vi "UseDeviceKey (with Device VIs).vi"() -> ()   [LabVIEW 2009]
panel:
  out "Device Count":i32
  out "Device Keys Out":string[](array[string])
  out "Output:":string
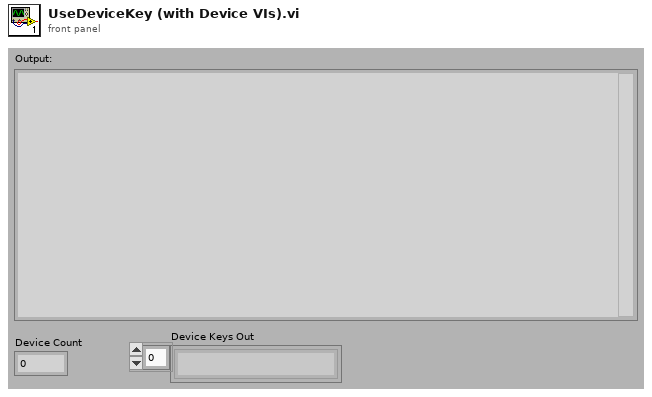
[diagram p1: front panel]
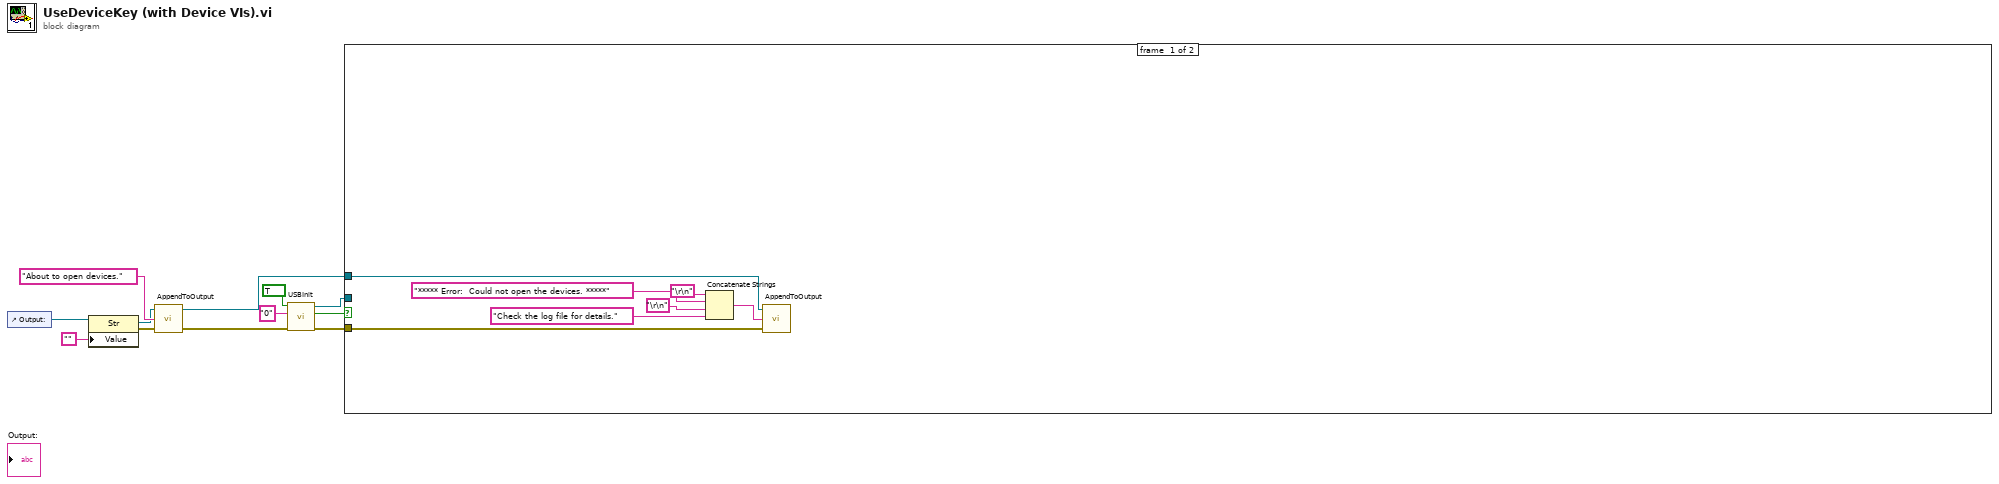
[diagram p0: block diagram]
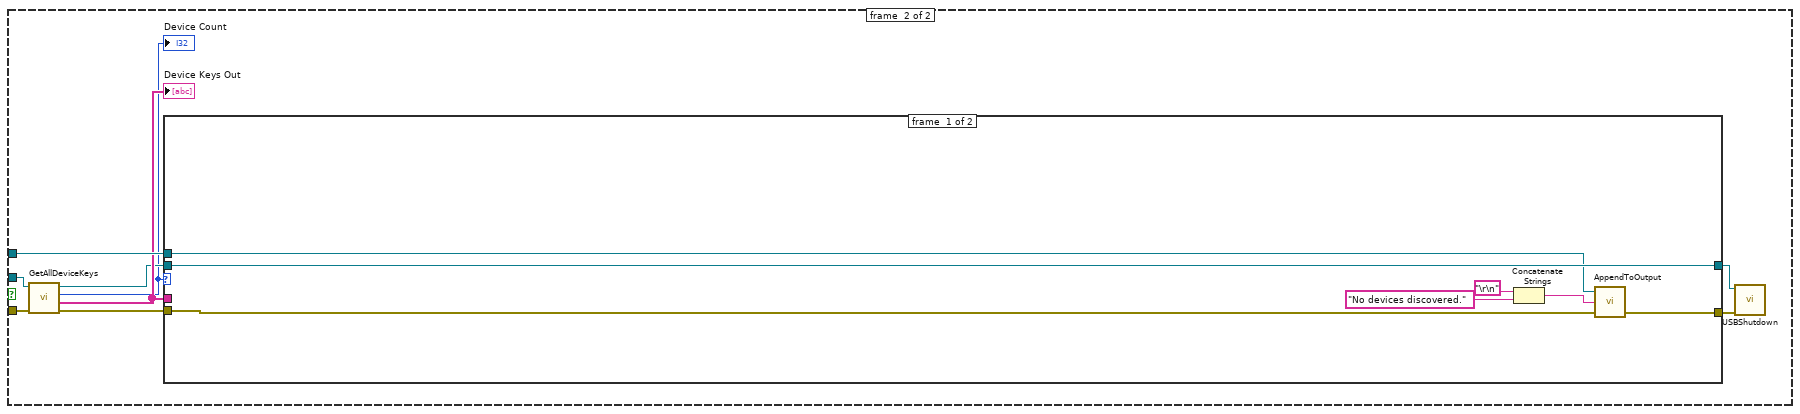
[diagram p2: hidden frame]
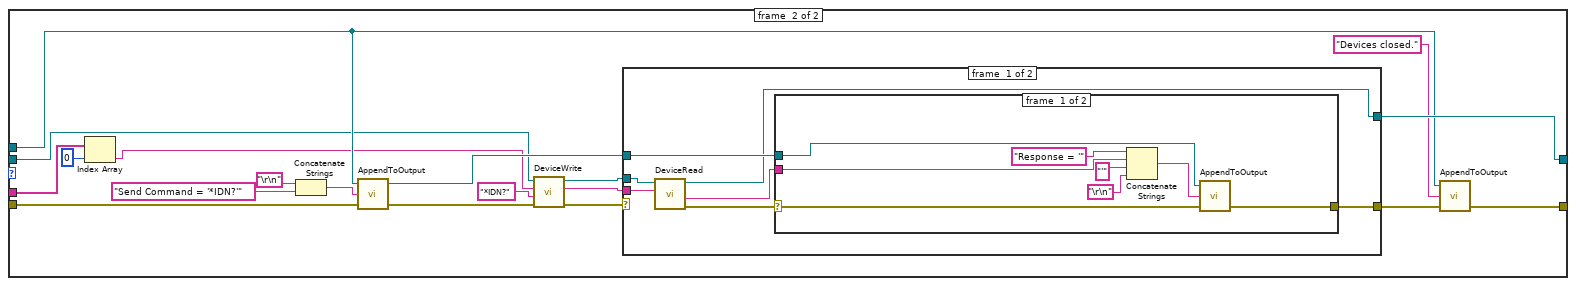
[diagram p3: hidden frame]
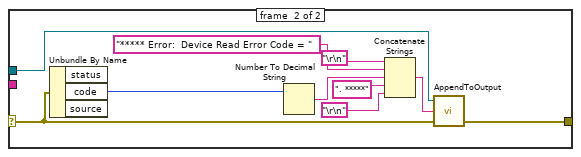
[diagram p4: hidden frame]
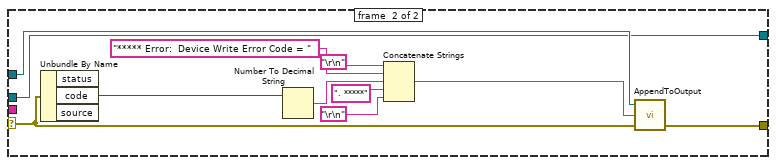
[diagram p5: hidden frame]
diagram:
  n1 = control-ref of="Output:"() -> (w10:refnum<vi>)
  n2 = property class="Str"(reference=w10, "Value"="") -> (reference out=w7:refnum<vi>, error out=w8:errorcluster)  [unwired: 1 in]
  n3 = call "AppendToOutput.vi"("error in"=w8, "Input String"="About to open devices.", "Output Refnum In"=w7) -> ("error out"=w4:errorcluster, "Output Refnum Out"=w11:refnum<vi>)  [unwired: 1 in]
  n4 = call "USBInit.vi"("error in (no error)"=w4, "Product ID"="0", "logging"=TRUE) -> ("error out"=w2:errorcluster, "Pass-Fail Status"=w3:bool, "USBLib Out"=w1:refnum<k24>)  [unwired: 2 in]
  n5 = case shown="True" w3 {
    tunnel: w11 -> [w19 w24]
    tunnel: w2 -> [w18 w25]
    tunnel: w1 -> [_ w26]
    frame #0 {
      n6 = Concatenate Strings("\r\n", "***** Error:  Could not open the devices. *****", "\r\n", "Check the log file for details.") -> (w14:string)
      n7 = call "AppendToOutput.vi"("error in"=w18, "Input String"=w14, "Output Refnum In"=w19) -> ()  [unwired: 1 in, 2 out]
    }
    frame #1 {
      n8 = call "GetAllDeviceKeys.vi"("error in (no error)"=w25, "USBLib In"=w26) -> ("error out"=w21:errorcluster, "Device Keys Out"=w23:string[], "Device Count"=w20:i32, "USBLib Out"=w22:refnum<k24>)  [unwired: 6 in]
      "Device Keys Out" <- w23
      "Device Count" <- w20
      n9 = case shown="1, Default" w20 {
        tunnel: [w32 w52] -> w28
        tunnel: [w35 w51] -> w27
        tunnel: w24 -> [w34 w50]
        tunnel: w23 -> [_ w44]
        tunnel: w22 -> [w35 w41]
        tunnel: w21 -> [w33 w40]
        frame #0 {
          n10 = Concatenate Strings("\r\n", "No devices discovered." ("Input String")) -> (w29:string)
          n11 = call "AppendToOutput.vi"("error in"=w33, "Input String"=w29, "Output Refnum In"=w34) -> ("error out"=w32:errorcluster)  [unwired: 1 in, 1 out]
        }
        frame #1 {
          n12 = Index Array(array=w44, index=0) -> (element=w42:string)
          n13 = Concatenate Strings("\r\n", "Send Command = '*IDN?'") -> (w36:string)
          n14 = call "AppendToOutput.vi"("error in"=w40, "Input String"=w36, "Output Refnum In"=w50) -> ("error out"=w49:errorcluster, "Output Refnum Out"=w54:refnum<vi>)  [unwired: 1 in]
          n15 = call "DeviceWrite.vi"("error in (no error)"=w49, "Command"="*IDN?" ("cmd"), "DeviceKey In"=w42, "USBLib In"=w41) -> ("error out"=w45:errorcluster, "DeviceKey Out"=w47:string, "USBLib Out"=w46:refnum<k24>)  [unwired: 1 in]
          n16 = case shown="No Error" w45 {
            selector: w45 -> [_ w81]
            tunnel: [w61 w84] -> w53
            tunnel: w54 -> [w60 w83]
            tunnel: w47 -> [w57 _]
            tunnel: [w59 w80] -> w51
            tunnel: w46 -> [w58 w80]
            frame #0 {
              n17 = call "DeviceRead.vi"("DeviceKey In"=w57, "USBLib In"=w58) -> ("error out"=w56:errorcluster, "Response"=w55:string, "USBLib Out"=w59:refnum<k24>)  [unwired: 2 in, 1 out]
              n18 = case shown="No Error" w56 {
                selector: w56 -> [w62 w70]
                tunnel: [w65 w72] -> w61
                tunnel: w60 -> [w64 w73]
                tunnel: w55 -> [w63 _]
                frame #0 {
                  n19 = Concatenate Strings("Response = '", w63, "'", "\r\n") -> (w66:string)
                  n20 = call "AppendToOutput.vi"("error in"=w62, "Input String"=w66, "Output Refnum In"=w64) -> ("error out"=w65:errorcluster)  [unwired: 1 in, 1 out]
                }
                frame #1 {
                  n21 = Unbundle By Name(w70) -> ("code"=w71:i32)  [unwired: 2 out]
                  n22 = Number To Decimal String(number=w71) -> (decimal integer string=w79:string)  [unwired: 1 in]
                  n23 = Concatenate Strings("\r\n", "***** Error:  Device Read Error Code = ", w79, ". *****", "\r\n") -> (w74:string)
                  n24 = call "AppendToOutput.vi"("error in"=w70, "Input String"=w74, "Output Refnum In"=w73) -> ("error out"=w72:errorcluster)  [unwired: 1 in, 1 out]
                }
              }
            }
            frame #1 {
              n25 = Unbundle By Name(w81) -> ("code"=w82:i32)  [unwired: 2 out]
              n26 = Number To Decimal String(number=w82) -> (decimal integer string=w86:string)  [unwired: 1 in]
              n27 = Concatenate Strings("\r\n", "***** Error:  Device Write Error Code = ", w86, ". *****", "\r\n") -> (w85:string)
              n28 = call "AppendToOutput.vi"("error in"=w81, "Input String"=w85, "Output Refnum In"=w83) -> ("error out"=w84:errorcluster)  [unwired: 1 in, 1 out]
            }
          }
          n29 = call "AppendToOutput.vi"("error in"=w53, "Input String"="Devices closed." ("string"), "Output Refnum In"=w50) -> ("error out"=w52:errorcluster)  [unwired: 1 in, 1 out]
        }
      }
      n30 = call "USBShutdown.vi"("error in (no error)"=w28, "USBLib In"=w27) -> ()  [unwired: 9 in, 1 out]
    }
  }
